vi "Main.vi"(8 "error in (no error)":errorcluster, 11 "Stop notifier":refnum<notifier>) -> (0 "error out":errorcluster)   [LabVIEW 2017, in "UI.lvlib"]
doc: "Module main"
uses:
  UI.lvlib
  ctl/StateData.ctl
  ctl/MainStates.ctl
  ctl/Price.ctl
  <vilib>/ErrorRing/Error Ring.xnode
  Error/Error.lvlib
panel:
  in  "Stop Button":bool
  out "Web":bool
  out "R":waveform(dbl)(graph)
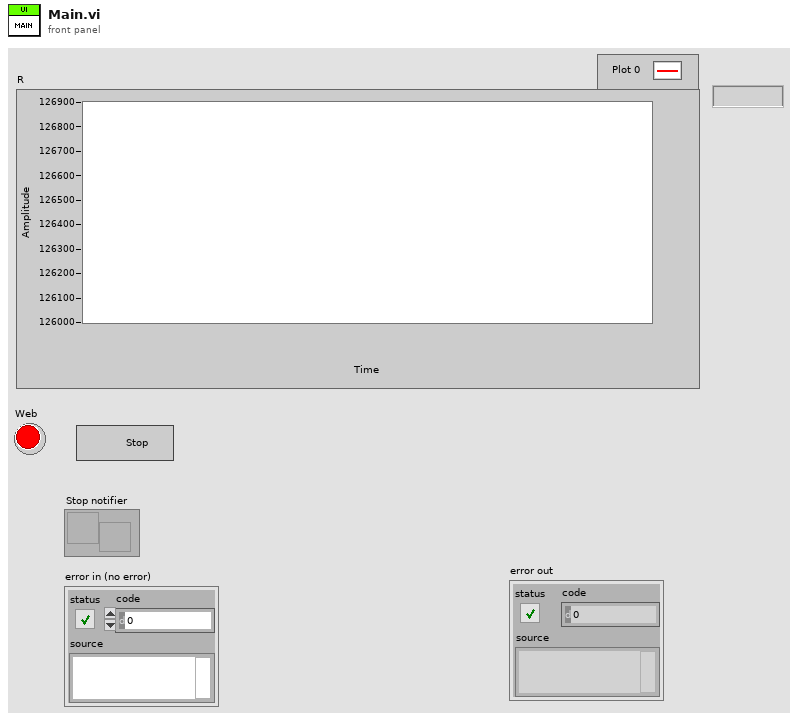
[diagram p1: front panel]
types:
  T1 = typedef "UI.lvlib/StateData.ctl" = cluster{"Blank":dbl}
  T2 = typedef "UI.lvlib/Price.ctl" = cluster{"USD":dbl, "Time Stamp":timestamp}
  T3 = typedef "UI.lvlib/MainStates.ctl" = enum16{"Timeout", "Error", "Exit", "Init", "UpdatePrice", "CloseAll"}
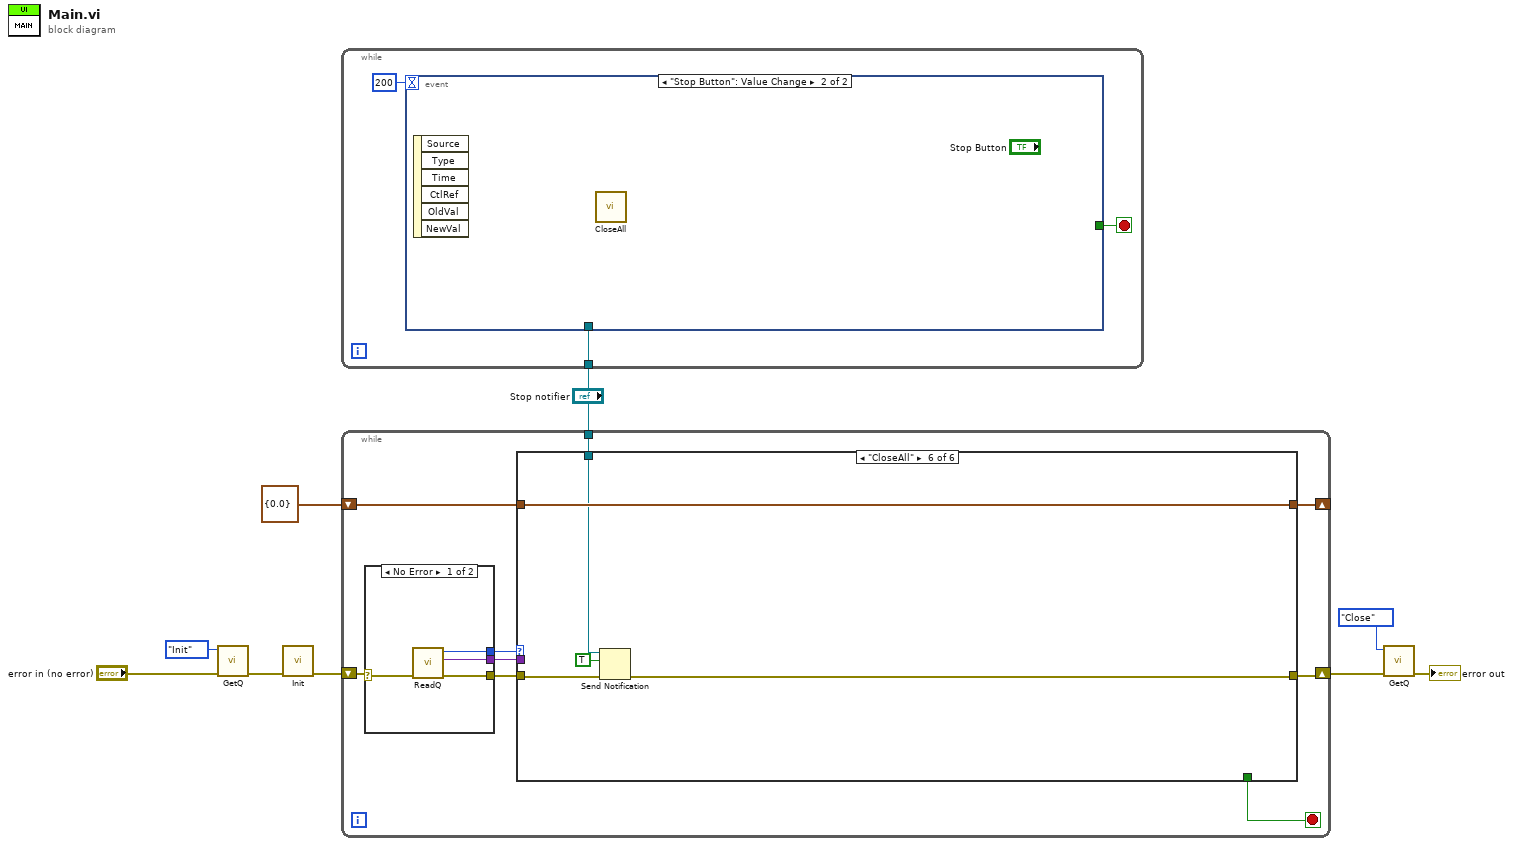
[diagram p0: block diagram]
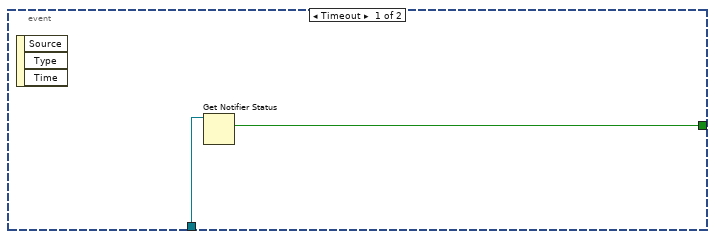
[diagram p2: hidden frame]
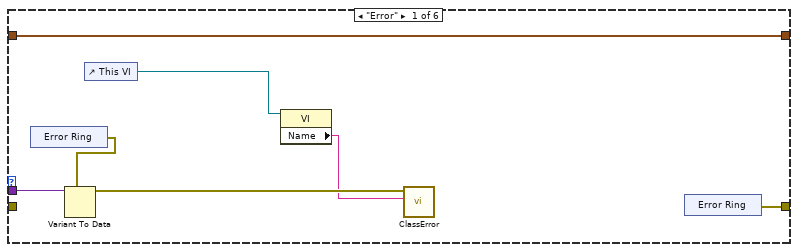
[diagram p3: hidden frame]
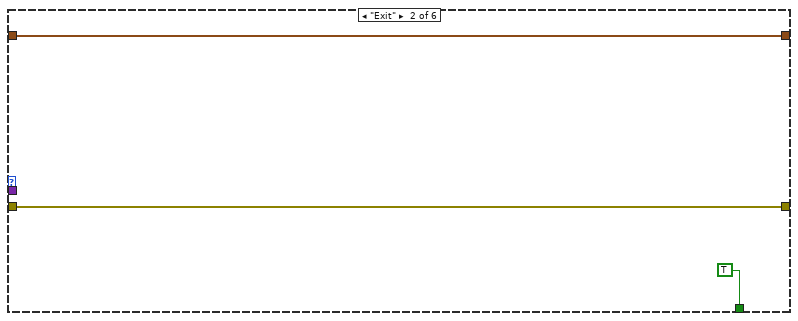
[diagram p4: hidden frame]
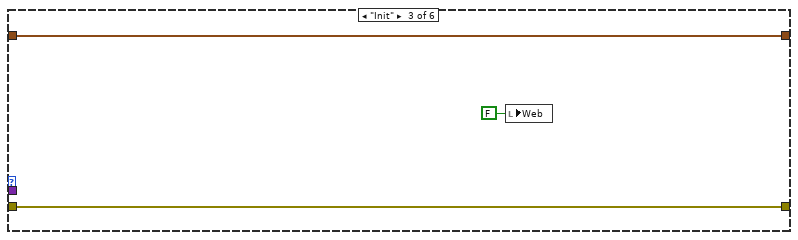
[diagram p5: hidden frame]
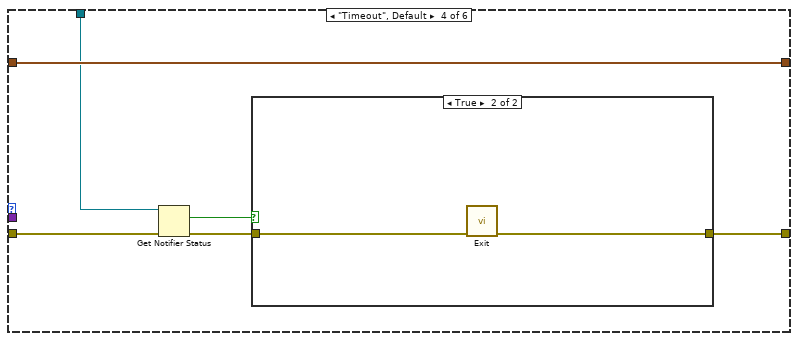
[diagram p6: hidden frame]
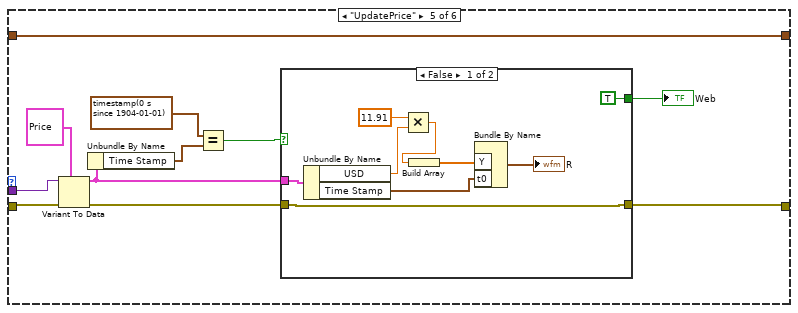
[diagram p8: hidden frame]
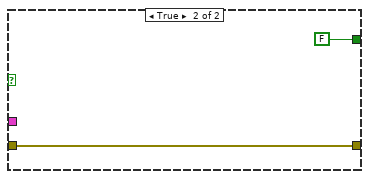
[diagram p9: hidden frame]
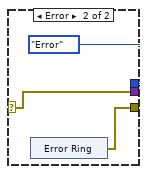
[diagram p10: hidden frame]
diagram:
  n1 = call "GetQ.vi"("error in (no error)"="error in (no error)", "Mode (Get)"=enum16{"Get", "Close", "Init"}."Init") -> ("error out"=w3:errorcluster)  [unwired: 8 in, 1 out]
  n2 = call "Init.vi"("error in (no error)"=w3) -> ("error out"=w2:errorcluster)  [unwired: 10 in]
  n3 = while {
    tunnel: "Stop notifier" -> [w11]
    stop <- w10 stop-if-true
    n4 = event shown="[1] \"Stop Button\": Value Change" {
      selector: _ -> [_ _]
      dyn-events: _ -> [_ _]
      timeout: 200 -> [_ _]
      tunnel: w11 -> [w14 _]
      tunnel: [w13 _] -> w10
      event Timeout {
        n5 = event-data() -> ()  [unwired: 1 in, 3 out]
        n6 = Get Notifier Status(notifier=w14) -> (current notification=w13:bool)  [unwired: 1 in, 4 out]
      }
      event "Stop Button": Value Change {
        n7 = event-data() -> ()  [unwired: 1 in, 6 out]
        n8 = call "CloseAll.vi"() -> ()  [unwired: 11 in, 1 out]
      }
    }
  }
  n9 = while {
    shift-right: [w19] -> w6
    shift-left: w2 -> [w23]
    shift-right: [w16] -> _
    shift-left: T1 {"Blank"=0.0} ("Cluster") -> [w17]
    tunnel: "Stop notifier" -> [w15]
    stop <- w18 stop-if-true
    n10 = case shown="No Error" w23 {
      selector: w23 -> [w78 w80]
      tunnel: [w77 MainStates."Error" ("State")] -> w22
      tunnel: [w76 w80] -> w21
      tunnel: [w75 w79] -> w20
      frame No Error {
        n11 = call "ReadQ.vi"("error in (no error)"=w78) -> ("error out"=w75:errorcluster, "Variant"=w76:variant, "State"=w77:T3)  [unwired: 8 in]
      }
      frame Error {
        n12 = xnode "Error Ring"() -> ("error out"=w79:errorcluster)
      }
    }
    n13 = case shown="\"CloseAll\"" w22 {
      tunnel: w21 -> [w30 _ _ _ w56 _]
      tunnel: w20 -> [_ w35 w38 w43 w57 w71]
      tunnel: [w29 w35 w38 w40 w49 w70] -> w19
      tunnel: [_ TRUE _ _ _ _] -> w18
      tunnel: w17 -> [w27 w33 w37 w44 w58 w74]
      tunnel: [w27 w33 w37 w44 w58 w74] -> w16
      tunnel: w15 -> [_ _ _ w42 _ w73]
      frame "Error" {
        n14 = xnode "Error Ring"() -> ("error out"=w28:errorcluster)
        n15 = Variant To Data(type=w28, Variant=w30) -> (data=w26:errorcluster)  [unwired: 1 in, 1 out]
        n16 = control-ref of="This VI"() -> (w25:refnum<vi>)
        n17 = property class="VI"(reference=w25) -> ("Name"=w24:string)  [unwired: 1 in, 2 out]
        n18 = call "ClassError.vi"("From"=w24, "error in"=w26) -> ()  [unwired: 9 in, 1 out]
        n19 = xnode "Error Ring"() -> ("error out"=w29:errorcluster)
      }
      frame "Exit" {
      }
      frame "Init" {
        n20 = local write "Web"(FALSE ("Web")) -> ()
      }
      frame "Timeout", Default {
        n21 = Get Notifier Status(notifier=w42, error in (no error)=w43) -> (current notification=w41:bool, error out=w39:errorcluster)  [unwired: 3 out]
        n22 = case shown="True" w41 {
          tunnel: [w45 w46] -> w40
          tunnel: w39 -> [w45 w47]
          frame False {
          }
          frame True {
            n23 = call "Exit.vi"("error in (no error)"=w47) -> ("error out"=w46:errorcluster)  [unwired: 10 in]
          }
        }
      }
      frame "UpdatePrice" {
        n24 = Variant To Data(error in=w57, type=T2 {"USD"=0.0, "Time Stamp"=timestamp(0 s since 1904-01-01)} ("Price"), Variant=w56) -> (data=w48:T2, error out=w51:errorcluster)
        n25 = Unbundle By Name(w48) -> ("Time Stamp"=w53:timestamp)
        n26 = Equal?(x=timestamp(0 s since 1904-01-01) ("Time Stamp"), y=w53) -> (x = y?=w52:bool)
        n27 = case shown="False" w52 {
          tunnel: w51 -> [w62 w68]
          tunnel: [TRUE ("Web") FALSE ("Web")] -> w50
          tunnel: [w62 w68] -> w49
          tunnel: w48 -> [w66 _]
          frame False {
            n28 = Unbundle By Name(w66) -> ("USD"=w61:dbl, "Time Stamp"=w65:timestamp)
            n29 = Multiply(x=11.91, y=w61) -> (x*y=w59:dbl)
            n30 = Build Array(w59) -> (w64:dbl[])
            n31 = Bundle By Name("Y"=w64, "t0"=w65) -> (→"R":waveform(dbl))  [unwired: 1 in]
          }
          frame True {
          }
        }
        "Web" <- w50
      }
      frame "CloseAll" {
        n32 = Send Notification(notification=TRUE, notifier=w73, error in (no error)=w71) -> (error out=w70:errorcluster)  [unwired: 1 out]
      }
    }
  }
  n33 = call "GetQ.vi"("error in (no error)"=w6, "Mode (Get)"=enum16{"Get", "Close", "Init"}."Close") -> ("error out"=→"error out":errorcluster)  [unwired: 8 in, 1 out]
